vi "RadWag Counting Pieces.vi"() -> ()   [LabVIEW 2016]
doc: "This VI is used to present how to configure balance operating mode on \"Parts Counting\" example."
uses:
  <instrlib>/RadWag balances and scales/RadWag balances and scales.lvlib
panel:
  in  "Single Piece Weight [g]":dbl=1.0
  out "Number of pieces":dbl
  in  "Stop":bool
  in  "VISA resource name":refnum<visa-resource-name>
  # "(c) 2014 Przemysłowy Instytut Automatyki i Pomiarów PIAP.  ALL RIGHTS RESERVED."
  # "Set weight of single piece\n before running this VI."
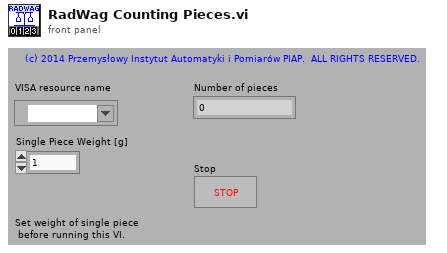
[diagram p1: front panel]
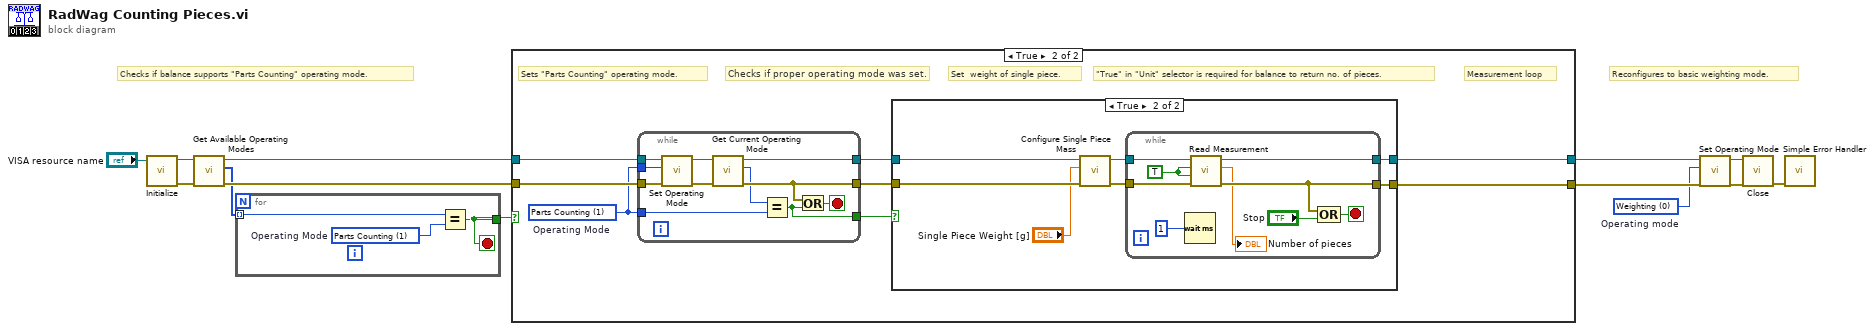
[diagram p0: block diagram]
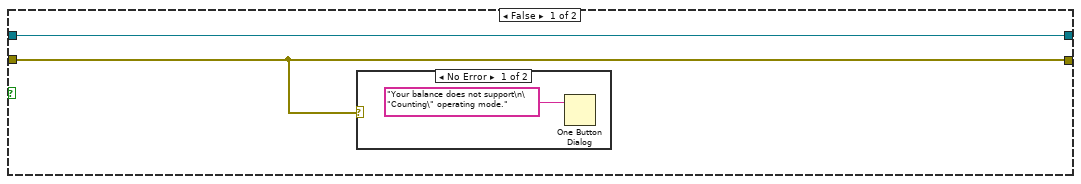
[diagram p2: hidden frame]
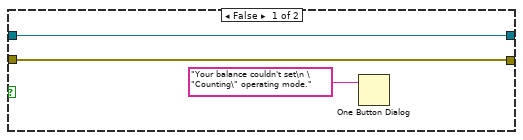
[diagram p4: hidden frame]
diagram:
  w3 = u16 0 items=["Weighting", "Counting", "Deviations", "Dosage", "Recipes", "Animals weighing", "Density", "Density of solids", "Density of liquids", "Maximum latch", "Addition", "Checkweighing", "Statistics", "Calibration of pipettes", "Differential weighing", "Statistical quality control (SQC)", "Product inspection", "Weight control (tableting)", "Drying", "Comparator", "Weighbridge"]  # Operating mode
  # "Reconfigures to basic weighting mode."
  # "Checks if balance supports \"Parts Counting\" operating mode."
  n1 = call <instrlib>:"Initialize.vi"("VISA resource name"="VISA resource name") -> ("error out"=w12:errorcluster, "VISA resource name out"=w13:refnum<visa-resource-name>)  [unwired: 9 in]
  n2 = call <instrlib>:"Get Available Operating Modes.vi"("error in (no error)"=w12, "VISA resource name"=w13) -> ("error out"=w9:errorcluster, "Operating Modes"=w8:i32[], "VISA resource name out"=w10:refnum<visa-resource-name>)  [unwired: 7 in]
  n3 = for {
    tunnel: w8 -> [w15] mode=indexing
    tunnel: [w16] -> w7
    stop <- w16 stop-if-true
    w14 = u16 1 items=["Weighing", "Parts Counting", "Deviations", "Dosing", "Formulas", "Animals Weighing", "Density", "Density of Solid Bodies", "Density of Liquids", "Peak Hold", "Totalizing", "Checkweighin", "Statistics", "Pipettes Calibration", "Differential weighing", "Statistical quality control (SQC)", "Product inspection", "Weight control (tableting)", "Drying", "Comparator", "Weighbridge"]  # Operating Mode
    n4 = Equal?(x=w15, y=w14) -> (x = y?=w16:bool)
  }
  n5 = case shown="True" w7 {
    tunnel: w10 -> [w18 w27]
    tunnel: w9 -> [w17 w26]
    tunnel: [w18 w25] -> w6
    tunnel: [w17 w24] -> w4
    frame False {
      n6 = case shown="No Error" w17 {
        frame No Error {
          n7 = One Button Dialog(message="Your balance does not support\n\"Counting\" operating mode.") -> ()  [unwired: 1 in, 1 out]
        }
        frame Error {
        }
      }
    }
    frame True {
      w20 = u16 1 items=["Weighing", "Parts Counting", "Deviations", "Dosing", "Formulas", "Animals Weighing", "Density", "Density of Solid Bodies", "Density of Liquids", "Peak Hold", "Totalizing", "Checkweighin", "Statistics", "Pipettes Calibration", "Differential weighing", "Statistical quality control (SQC)", "Product inspection", "Weight control (tableting)", "Drying", "Comparator", "Weighbridge"]  # Operating Mode
      # "\"True\" in \"Unit\" selector is required for balance to return no. of pieces."
      # "Measurement loop"
      # "Set  weight of single piece."
      # "Checks if proper operating mode was set."
      # "Sets \"Parts Counting\" operating mode."
      n8 = while {
        tunnel: w27 -> [w38]
        tunnel: w26 -> [w37]
        tunnel: [w35] -> w23
        tunnel: [w32] -> w22
        tunnel: [w31] -> w21
        tunnel: w20 -> [w30]
        tunnel: w20 -> [w29]
        stop <- w33 stop-if-true
        n9 = call <instrlib>:"Set Operating Mode.vi"("error in (no error)"=w37, "Operating mode (0: Weighting)"=w30, "VISA resource name"=w38) -> ("error out"=w34:errorcluster, "VISA resource name out"=w36:refnum<visa-resource-name>)  [unwired: 7 in]
        n10 = call <instrlib>:"Get Current Operating Mode.vi"("error in (no error)"=w34, "VISA resource name"=w36) -> ("error out"=w32:errorcluster, "Operating Mode"=w28:i32, "VISA resource name out"=w35:refnum<visa-resource-name>)  [unwired: 7 in]
        n11 = Equal?(x=w28, y=w29) -> (x = y?=w31:bool)
        n12 = Or(x=w32, y=w31) -> (x .or. y?=w33:bool)
      }
      n13 = case shown="True" w21 {
        tunnel: w23 -> [w41 w48]
        tunnel: [w41 w45] -> w25
        tunnel: [w40 w44] -> w24
        tunnel: w22 -> [w40 w43]
        frame False {
          n14 = One Button Dialog(message="Your balance couldn't set\n \"Counting\" operating mode.") -> ()  [unwired: 1 in, 1 out]
        }
        frame True {
          n15 = call <instrlib>:"Configure Single Piece Mass.vi"("error in (no error)"=w43, "Single Piece Weight [g]"="Single Piece Weight [g]", "VISA resource name"=w48) -> ("error out"=w46:errorcluster, "VISA resource name out"=w47:refnum<visa-resource-name>)  [unwired: 7 in]
          n16 = while {
            tunnel: w47 -> [w54]
            tunnel: w46 -> [w51]
            tunnel: [w53] -> w45
            tunnel: [w52] -> w44
            stop <- w57 stop-if-true
            w50 = TRUE ("Base unit (F)/ Acctual unit (T)")
            n17 = Wait (ms)(milliseconds to wait=u32 1) -> ()  [unwired: 1 out]
            n18 = call <instrlib>:"Read Measurement.vi"("error in (no error)"=w51, "Actual Unit (F: Base unit)"=w50, "Immediately  (F: Wait for stable result)"=w50, "VISA resource name"=w54) -> ("error out"=w52:errorcluster, "Value"=→"Number of pieces":dbl, "VISA resource name out"=w53:refnum<visa-resource-name>)  [unwired: 3 in, 2 out]
            n19 = Compound Arithmetic op=OR(w52, "Stop") -> (w57:bool)
          }
        }
      }
    }
  }
  n20 = call <instrlib>:"Set Operating Mode.vi"("error in (no error)"=w4, "Operating mode (0: Weighting)"=w3, "VISA resource name"=w6) -> ("error out"=w2:errorcluster, "VISA resource name out"=w5:refnum<visa-resource-name>)  [unwired: 7 in]
  n21 = call <instrlib>:"Close.vi"("error in (no error)"=w2, "VISA resource name"=w5) -> ("error out"=w1:errorcluster)  [unwired: 9 in]
  n22 = call <vilib>:"Simple Error Handler.vi"("error in (no error)"=w1) -> ()  [unwired: 4 in, 5 out]
